vi "TDMS文件名.vi"() -> ()   [LabVIEW 2013]
panel:
  in  "TDMS文件名":string
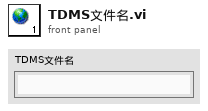
[diagram p1: front panel]
diagram:
